vi "pumpsec_09_4.vi"(0 "reset":i32, 1 "master":i32, 4 "manual":i32, 5 "pause":i32, 7 "Port":i32=10, 8 "pump_type":i32, 9 "port, Reglo D":i32, 14 "Target":dbl[](array[numeric])=[10.0, 2.0, 0.0, 0.0, 0.0, 0.0, 0.0, 0.0, 0.0, 0.0], 16 "fr_manual":dbl, 17 "Time":dbl[](array[numeric])=[4.0, 2.0, 0.0, 0.0, 0.0, 0.0, 0.0, 0.0, 0.0, 0.0]) -> (11 "time_to_target":dbl, 12 "step_fr":dbl, 13 "amount_step":dbl, 15 "Reglo D":dbl, 19 "reset_out":dbl, 20 "Scale":dbl, 21 "mA":dbl format="%#_2g", 23 "elapsed_step":dbl, 24 "Scale actual":dbl, 25 "params":dbl[](array[numeric]), 27 "PAM":dbl)   [LabVIEW 2015]
uses:
  BERTTA.dll
panel:
  out "amount_step_previous":dbl
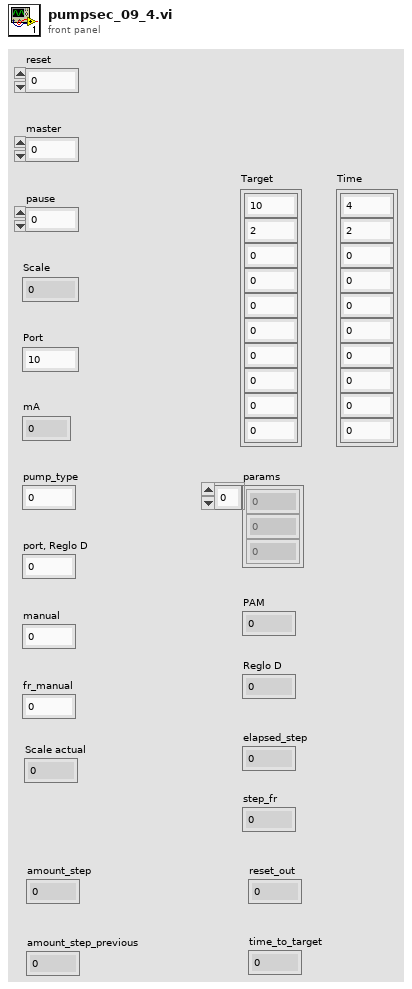
[diagram p1: front panel]
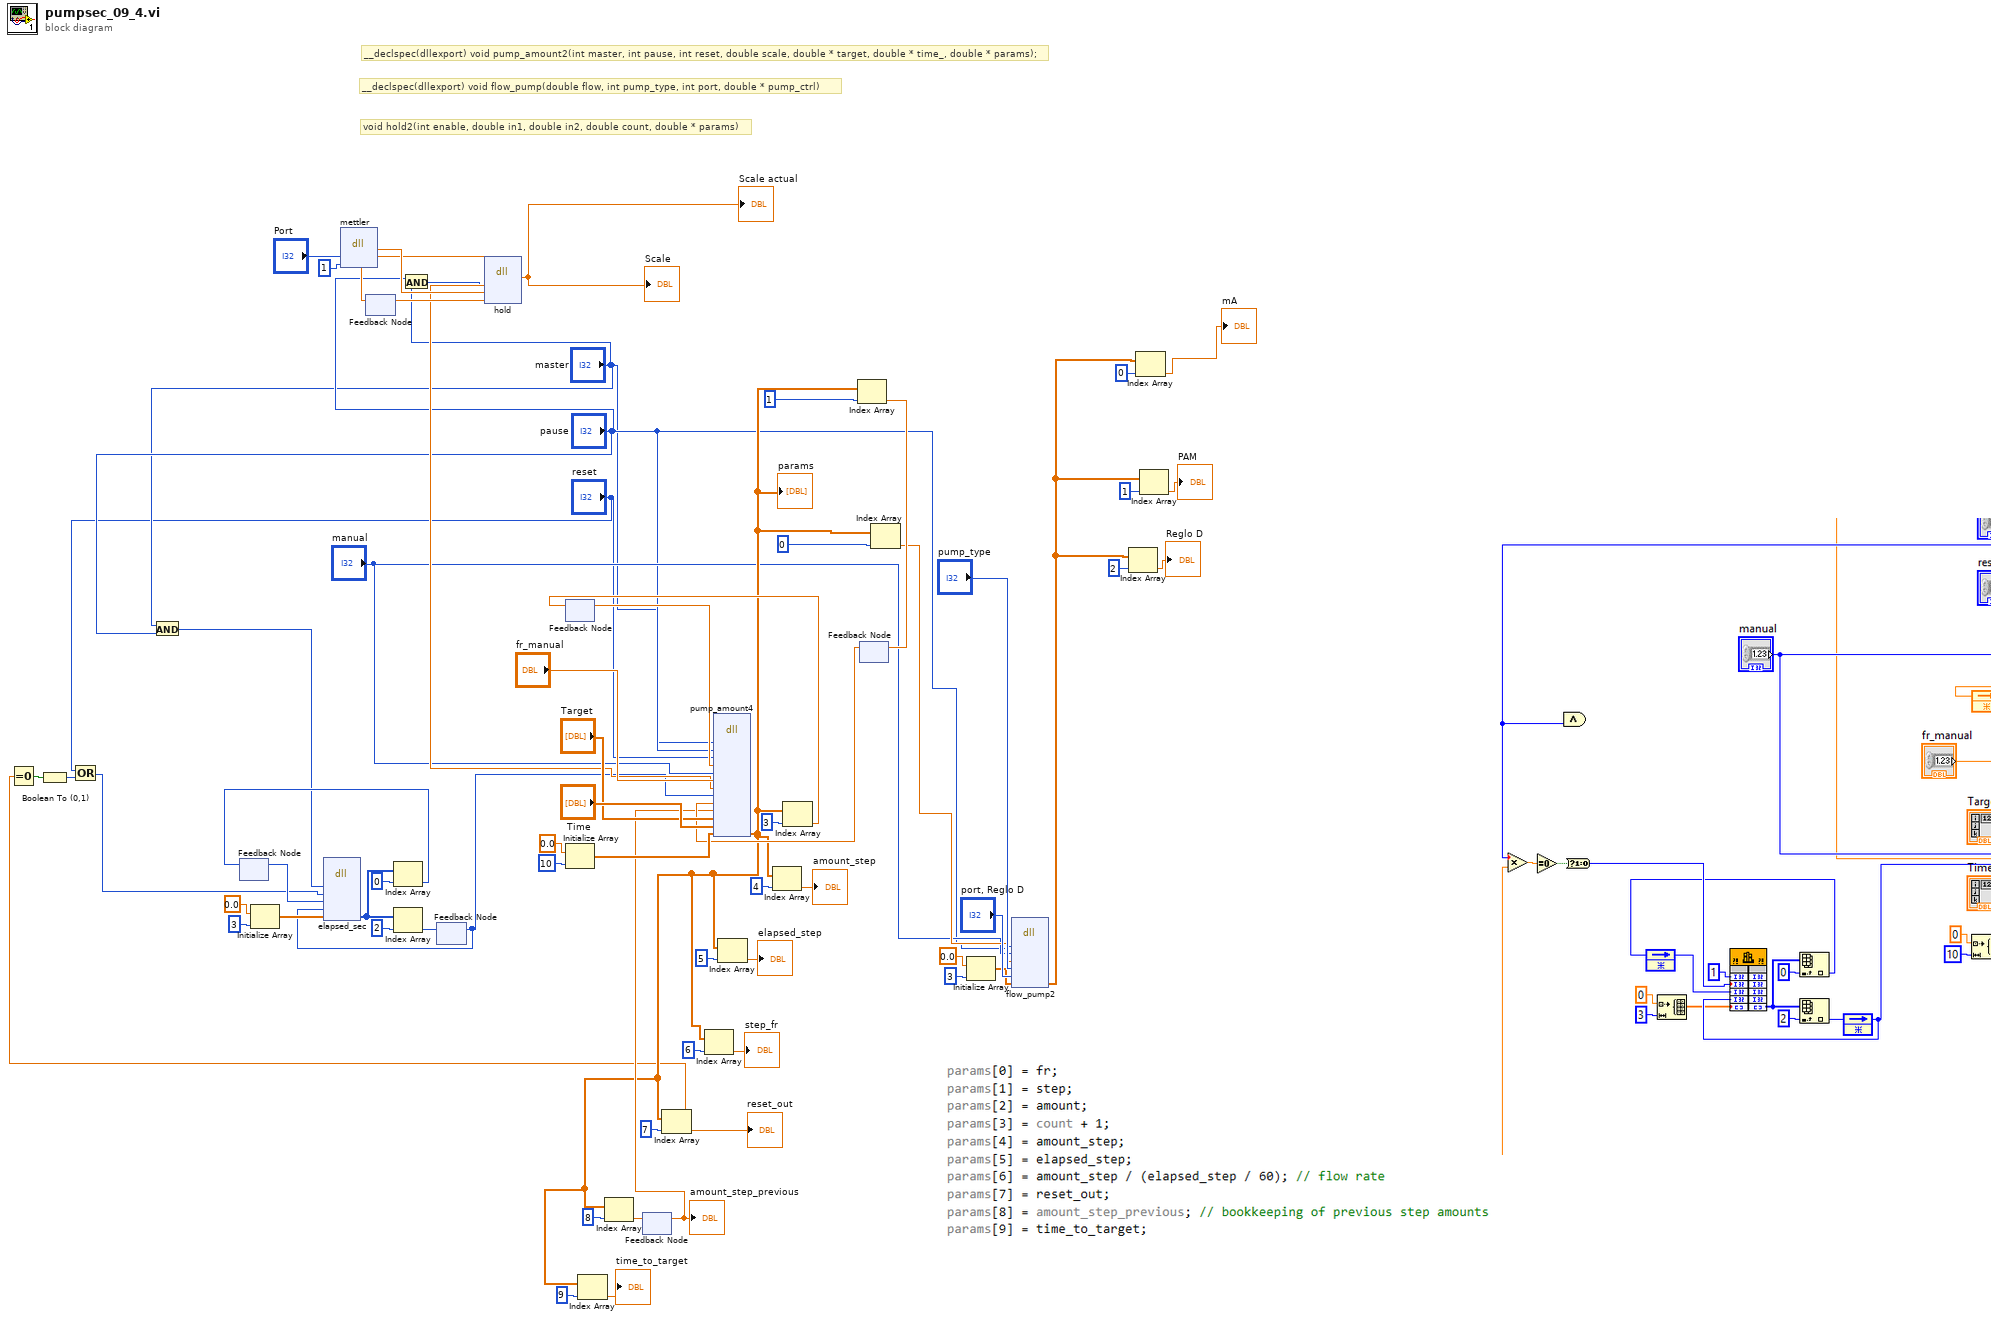
[diagram p0: block diagram]
diagram:
  # "void hold2(int enable, double in1, double in2, double count, double * params)"
  # "__declspec(dllexport) void flow_pump(double flow, int pump_type, int port, double * pump_ctrl)"
  # "__declspec(dllexport) void pump_amount2(int master, int pause, int reset, double scale, double * target, double * time_, double * params);"
  n1 = And(x="master", y="pause") -> (x .and. y?=w6:i32)
  n2 = feedback #1() -> (w19:i32)  [unwired: 1 in]
  n3 = Initialize Array(0.0 ("element"), 3 ("dimension size")) -> (w23:dbl[])
  n4 = dll-call lib="C:/Users/shresplab/OneDrive - Kemira Oyj/Documents/Visual Studio 2017/Projects/Bertta/BERTTA/x64/Debug/BERTTA.dll" fn="mettler"("port"="Port", "msg"=1) -> ("return type"=w43:dbl)  [unwired: 5 in, 2 out]
  n5 = feedback #2() -> (w42:dbl)  [unwired: 1 in]
  n6 = And(x="pause", y="master") -> (x .and. y?=w40:i32)
  n7 = feedback #3() -> (w17:i32)  [unwired: 1 in]
  n8 = dll-call lib="C:/Users/shresplab/OneDrive - Kemira Oyj/Documents/Visual Studio 2017/Projects/Bertta/BERTTA/x64/Debug/BERTTA.dll" fn="hold"("enable"=w40, "in1"=w43, "in2"=w42) -> ("return type"=w41:dbl)  [unwired: 6 in, 2 out]
  "Scale" <- w41
  "Scale actual" <- w41
  n9 = feedback-in #2(w41) -> ()
  n10 = feedback #4() -> (w37:dbl)  [unwired: 1 in]
  n11 = Initialize Array(0.0 ("element"), 10 ("dimension size")) -> (w50:dbl[])
  n12 = feedback #5() -> (w14:dbl)  [unwired: 1 in]
  "amount_step_previous" <- w14
  n13 = feedback #6() -> (w27:dbl)  [unwired: 1 in]
  n14 = dll-call lib="C:/Users/shresplab/OneDrive - Kemira Oyj/Documents/Visual Studio 2017/Projects/Bertta/BERTTA/x64/Debug/BERTTA.dll" fn="pump_amount4"("master"="master", "pause"="pause", "reset"="reset", "count"=w37, "manual"="manual", "fr_manual"="fr_manual", "scale"=w41, "elapsed"=w17, "step_previous"=w27, "amount_step_previous"=w14, "target"="Target", "time_"="Time", "params"=w50) -> ("params"=w11:dbl[])  [unwired: 16 in, 2 out]
  "params" <- w11
  n15 = Index Array(array=w11, index=9) -> (element=→"time_to_target":dbl)
  n16 = Index Array(array=w11, index=8) -> (element=w15:dbl)
  n17 = feedback-in #5(w15) -> ()
  n18 = Index Array(array=w11, index=7) -> (element=w3:dbl)
  "reset_out" <- w3
  n19 = Equal To 0?(x=w3) -> (x = 0?=w2:bool)
  n20 = Boolean To (0,1)(Boolean=w2) -> (0, 1=w1:i16)
  n21 = Or(x="reset", y=w1) -> (x .or. y?=w5:i32)
  n22 = dll-call lib="C:/Users/shresplab/OneDrive - Kemira Oyj/Documents/Visual Studio 2017/Projects/Bertta/BERTTA/x64/Debug/BERTTA.dll" fn="elapsed_sec"("enable"=w6, "reset"=w5, "last_time"=w19, "elapsed_last"=w17, "params"=w23) -> ("params"=w21:i32[])  [unwired: 8 in, 2 out]
  n23 = Index Array(array=w21, index=0) -> (element=w20:i32)
  n24 = feedback-in #1(w20) -> ()
  n25 = Index Array(array=w21, index=2) -> (element=w18:i32)
  n26 = feedback-in #3(w18) -> ()
  n27 = Index Array(array=w11, index=6) -> (element=→"step_fr":dbl)
  n28 = Index Array(array=w11, index=5) -> (element=→"elapsed_step":dbl)
  n29 = Index Array(array=w11, index=4) -> (element=→"amount_step":dbl)
  n30 = Index Array(array=w11, index=3) -> (element=w38:dbl)
  n31 = feedback-in #4(w38) -> ()
  n32 = Index Array(array=w11, index=1) -> (element=w28:dbl)
  n33 = feedback-in #6(w28) -> ()
  n34 = Index Array(array=w11, index=0) -> (element=w13:dbl)
  n35 = Initialize Array(0.0 ("element"), 3 ("dimension size")) -> (w55:dbl[])
  n36 = dll-call lib="C:/Users/shresplab/OneDrive - Kemira Oyj/Documents/Visual Studio 2017/Projects/Bertta/BERTTA/x64/Debug/BERTTA.dll" fn="flow_pump2"("enable"="pause", "manual"="manual", "flow"=w13, "pump_type"="pump_type", "port"="port, Reglo D", "pump_ctrl"=w55) -> ("pump_ctrl"=w46:dbl[])  [unwired: 9 in, 2 out]
  n37 = Index Array(array=w46, index=2) -> (element=→"Reglo D":dbl)
  n38 = Index Array(array=w46, index=0) -> (element=→"mA":dbl)
  n39 = Index Array(array=w46, index=1) -> (element=→"PAM":dbl)
